vi "2-Ch Optical Density.vi"(0 "Detuning":dbl[unit]=10000000.0, 5 "Linewidth":dbl[unit]=5234000.0, 7 "data":dbl[][](array[numeric]), 9 "Upper Threshold (% of Max)":dbl=80.0, 11 "Lower Threshold (% of Min)":dbl=120.0) -> (1 "Upper Voltage Threshold Reference":dbl, 2 "Upper Voltage Threshold Signal 1":dbl, 3 "Upper Voltage Threshold Signal 2":dbl, 10 "Optical Density 1":dbl, 12 "Lower Voltage Threshold Reference":dbl, 13 "Lower Voltage Threshold Signal 1":dbl, 14 "Lower Voltage Threshold Signal 2":dbl, 15 "Optical Density 2":dbl)   [LabVIEW 2009]
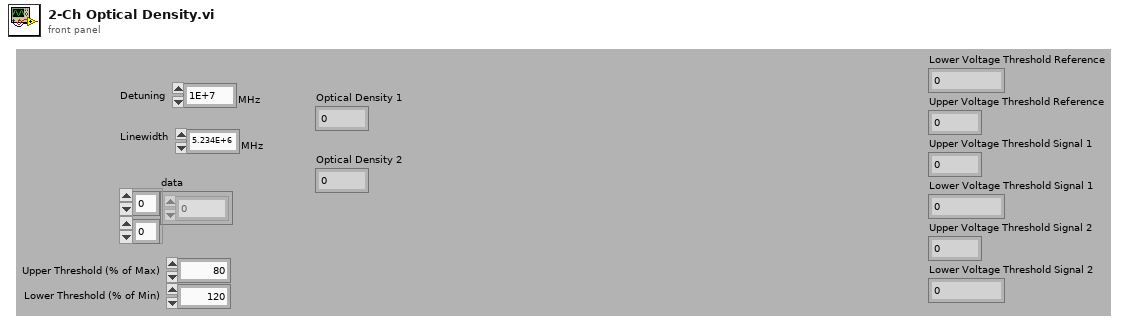
[diagram p1: front panel]
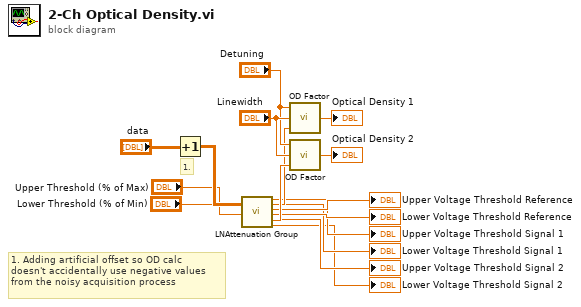
[diagram p0: block diagram]
diagram:
  # "1."
  # "1. Adding artificial offset so OD calc\ndoesn't accidentally use negative values \nfrom the noisy acquisition process"
  n1 = Increment(x="data") -> (x+1=w9:dbl[][])
  n2 = call "LNAttenuation Group.vi"("Upper Threshold (% of Max)"="Upper Threshold (% of Max)", "data"=w9, "Lower Threshold (% of Min)"="Lower Threshold (% of Min)") -> ("LN Attenuation1"=w11:dbl, "LN Attenuation 2"=w14:dbl, "Upper Voltage Threshold Channel 1"=→"Upper Voltage Threshold Signal 1":dbl, "Lower Voltage Threshold Channel 1"=→"Lower Voltage Threshold Signal 1":dbl, "Upper Voltage Threshold Reference"=→"Upper Voltage Threshold Reference":dbl, "Lower Voltage Threshold Reference"=→"Lower Voltage Threshold Reference":dbl, "Upper Voltage Threshold Signal 2"=→"Upper Voltage Threshold Signal 2":dbl, "Lower Voltage Threshold Signal 2"=→"Lower Voltage Threshold Signal 2":dbl)  [unwired: 9 in]
  n3 = call "OD Factor.vi"("LNAttenuation"=w11, "Linewidth"="Linewidth", "Detuning"="Detuning") -> ("Optical Density"=→"Optical Density 1":dbl)
  n4 = call "OD Factor.vi"("LNAttenuation"=w14, "Linewidth"="Linewidth", "Detuning"="Detuning") -> ("Optical Density"=→"Optical Density 2":dbl)
